vi "ClusterDemo-BinaryConversion.vi"() -> ()   [LabVIEW 2019]
panel:
  out "Numeric Value":dbl
  out "Input Cluster 2":cluster{"1":bool, "2":bool, "4":bool, "8":bool}
  in  "Input Cluster":cluster{"1":bool, "2":bool, "4":bool, "8":bool}
  # "Binary to Decimal Number Converter"
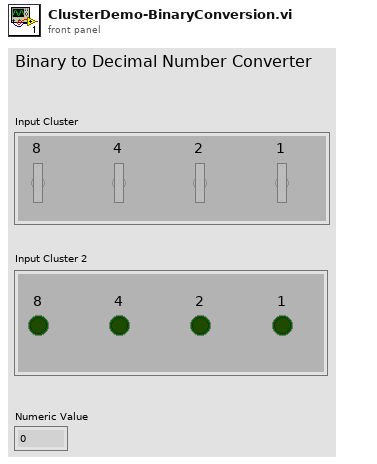
[diagram p1: front panel]
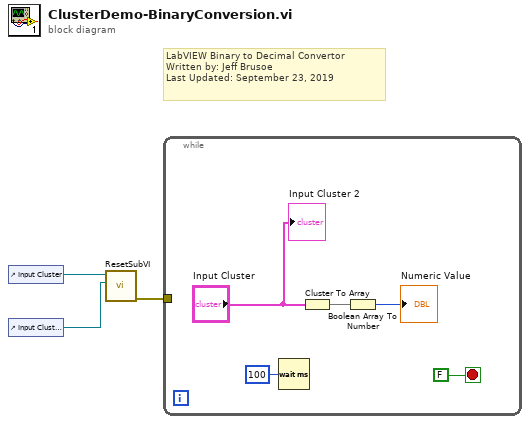
[diagram p0: block diagram]
diagram:
  # "LabVIEW Binary to Decimal Convertor\nWritten by: Jeff Brusoe\nLast Updated: September 23, 2019"
  n1 = control-ref of="Input Cluster"() -> (w2:refnum<vi>)
  n2 = control-ref of="Input Cluster 2"() -> (w1:refnum<vi>)
  n3 = call "ResetSubVI.vi"("Clust Refnum in"=w1, "Cluster in"=w2) -> ("error out"=w3:errorcluster)  [unwired: 9 in]
  n4 = while {
    tunnel: w3 -> [_]
    stop <- FALSE stop-if-true
    n5 = Wait (ms)(milliseconds to wait=u32 100) -> ()  [unwired: 1 out]
    n6 = Cluster To Array(cluster="Input Cluster") -> (array=w5:bool[])
    n7 = Boolean Array To Number(Boolean array=w5) -> (number=→"Numeric Value":u32)
    "Input Cluster 2" <- "Input Cluster"
  }
